vi "TestCompile.vi"() -> ()   [LabVIEW 2015]
panel:
  out "x*2^n":i16
  in  "n":i16
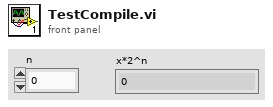
[diagram p1: front panel]
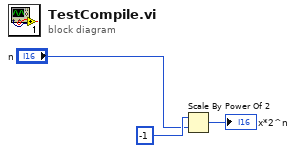
[diagram p0: block diagram]
diagram:
  n1 = Scale By Power Of 2(n=-1 ("x"), x="n") -> (x*2^n=→"x*2^n":i16)
